vi "g_SV_Connect_ALB.vi"(7 "Action":enum16{"read", "write"}(ring), 10 "Connect in":bool) -> (2 "Connected":bool)   [LabVIEW 2017]
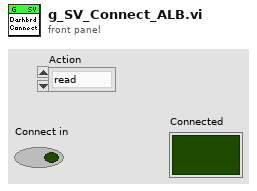
[diagram p1: front panel]
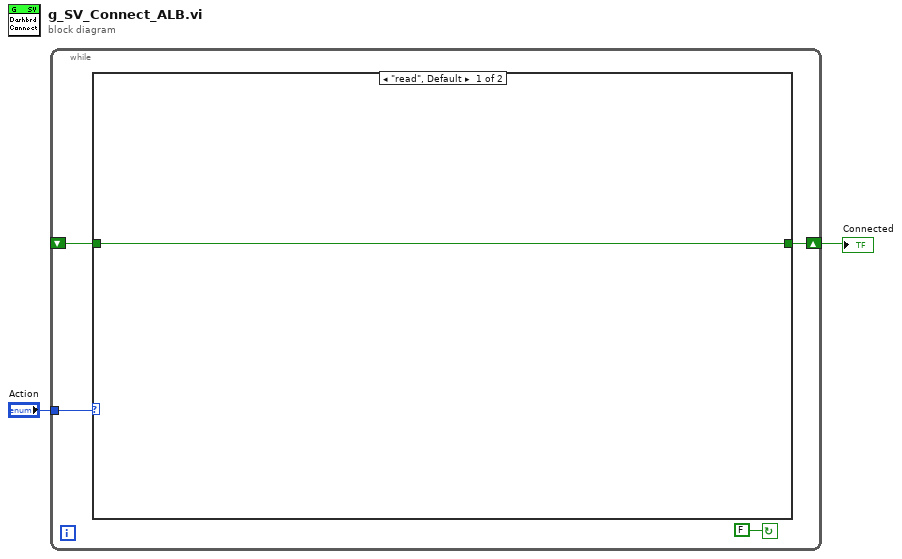
[diagram p0: block diagram]
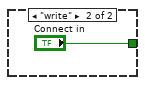
[diagram p2: hidden frame]
diagram:
  n1 = while {
    tunnel: "Action" -> [w5]
    shift-right: [w4] -> w1
    shift-left: _ -> [w3]
    stop <- FALSE continue-if-true
    n2 = case shown="\"read\", Default" w5 {
      tunnel: [w7 "Connect in"] -> w4
      tunnel: w3 -> [w7 _]
      frame "read", Default {
      }
      frame "write" {
      }
    }
  }
  "Connected" <- w1
